vi "Get Reduce Motor Torque.vi"(4 "error in (no error)":errorcluster, 6 "Axis (1)":i32=1 min=1 max=3, 7 "VISA resource name":refnum<visa-resource-name>) -> (0 "error out":errorcluster, 2 "Motor Current Reduced (%)":dbl format="%.4g", 3 "VISA resource name out":refnum<visa-resource-name>)   [LabVIEW 2010, in "Newport ESP301.lvlib"]
doc: "Reads the torque reduction setting for the specified axis."
uses:
  <userlib>/Newport ESP301/Newport ESP301.lvlib
panel:
  out "delay (ms)":i32
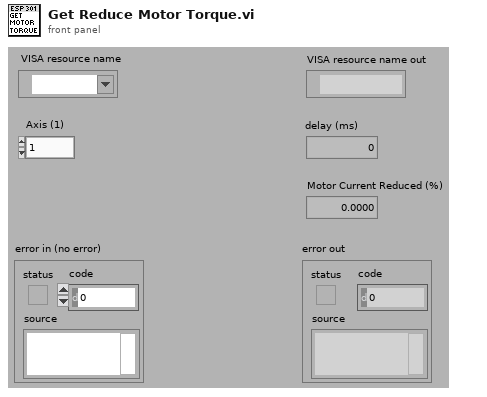
[diagram p1: front panel]
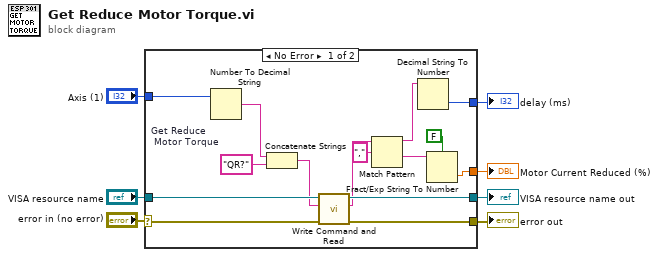
[diagram p0: block diagram]
diagram:
  n1 = case shown="No Error" "error in (no error)" {
    selector: "error in (no error)" -> [w19 w24]
    tunnel: [w21 w24] -> w7
    tunnel: "VISA resource name" -> [w22 w23]
    tunnel: [w20 w23] -> w6
    tunnel: [w18 _] -> w3
    tunnel: "Axis (1)" -> [w15 _]
    tunnel: [w9 _] -> w1
    frame No Error {
      w17 = "QR?"  # Get Reduce  Motor Torque
      n2 = Number To Decimal String(number=w15) -> (decimal integer string=w16:string)  [unwired: 1 out]
      n3 = Concatenate Strings(w16, w17) -> (w14:string)
      n4 = call <userlib>:"Write Command and Read.vi"("error in (no error)"=w19, "Command"=w14, "VISA resource name"=w22) -> ("error out"=w21:errorcluster, "Returned string"=w12:string, "VISA resource name out"=w20:refnum<visa-resource-name>)  [unwired: 2 in, 2 out]
      n5 = Match Pattern(string=w12, regular expression="," ("expression régulière")) -> (before substring=w8:string, after substring=w10:string)  [unwired: 1 in, 2 out]
      n6 = Decimal String To Number(string=w8) -> (number=w9:i32)  [unwired: 2 in, 1 out]
      n7 = Fract/Exp String To Number(use system decimal point (T)=FALSE ("utiliser le séparateur décimal du système (V)"), string=w10) -> (number=w18:dbl)  [unwired: 3 out]
    }
    frame Error {
    }
  }
  "error out" <- w7
  "VISA resource name out" <- w6
  "Motor Current Reduced (%)" <- w3
  "delay (ms)" <- w1
